vi "ndipolaris Measurement Example.vi"() -> ()   [LabVIEW 2013]
doc: "This example shows how to use the driver's VI's to set up the Polaris and acquire transformations. For this example, all wired tools are activated and one wireless tool is activated."
panel:
  out "Front View (YX)":cluster{dbl, dbl}[](graph)
  out "Left Side View (ZX)":cluster{dbl, dbl}[](graph)
  out "Top View (YZ)":cluster{dbl, dbl}[](graph)
  out "Current Transformations":T1(array[cluster])
  in  "Track Stray Markers? (F:No)":bool
  in  "VISA resource name":refnum<visa-resource-name>="COM1"
  in  "Reset? (T:Yes)":bool=TRUE
  in  "Track Outside Measurement Volume? (F:No)":bool
  in  "Location of ROM File for Tool":path=path "C:/Program Files/Northern Digital Inc/8700248.rom"
  in  "Serial Configuration":T2={"Baud Rate (9600)"=9600, "Flow Control (0:None)"=0, "Parity"=0, "Data Bits"=8, "Stop Bits"=10} {"Stop Bits" items=["1.0"=10, "2.0"=20]; "Parity" items=["None", "Odd", "Even"]; "Flow Control (0:None)" items=["None", "XON/XOFF"]; "Baud Rate (9600)" items=["9600"=9600, "14.4k"=14400, "19.2k"=19200, "38.4k"=38400, "57.6k "=57600, "115.2k"=115200]}
  in  "STOP":bool
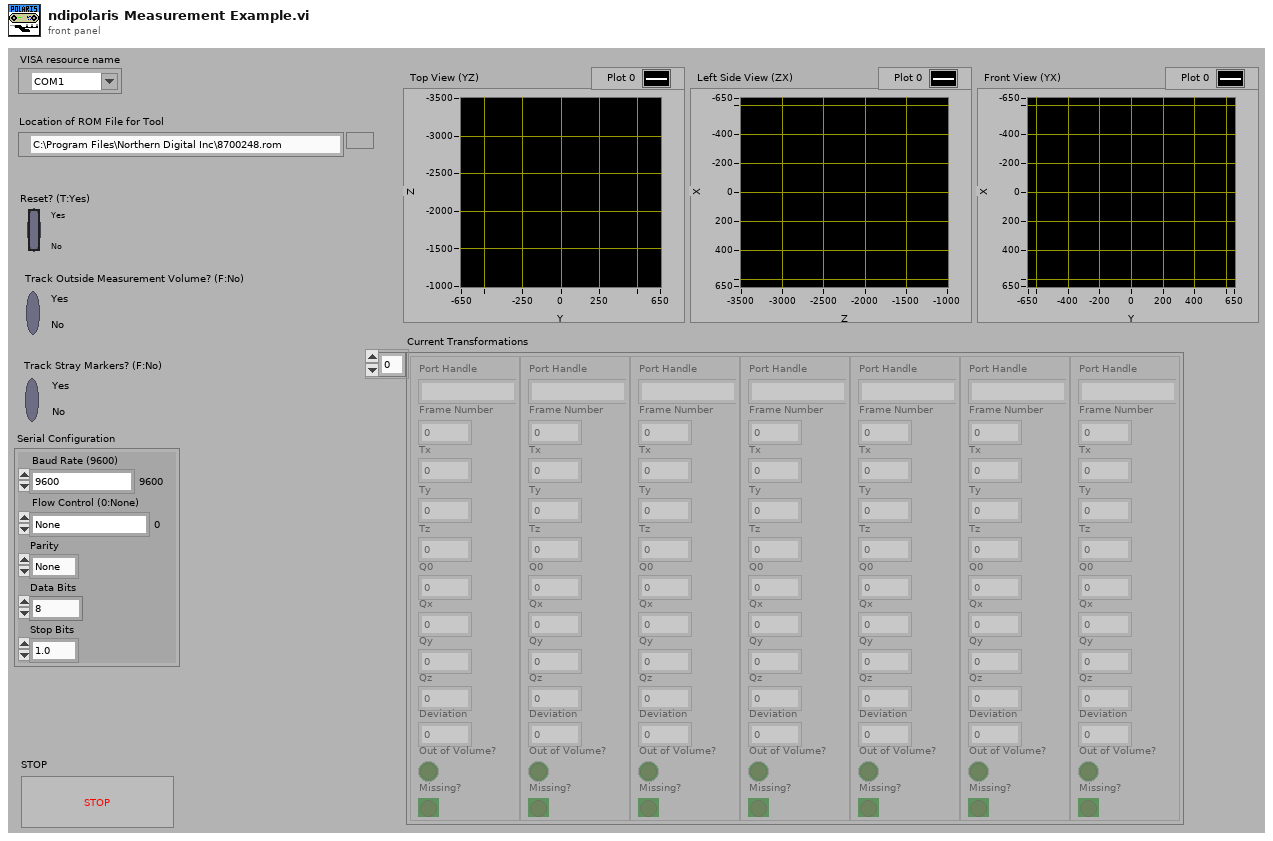
[diagram p1: front panel]
types:
  T1 = cluster{"Port Handle":string, "Frame Number":u32, "Tx":dbl, "Ty":dbl, "Tz":dbl, "Q0":dbl, "Qx":dbl, "Qy":dbl, "Qz":dbl, "Deviation":dbl, "Missing?":bool, "Out of Volume?":bool}[]
  T2 = cluster{"Baud Rate (9600)":u32, "Flow Control (0:None)":u16, "Parity":u16, "Data Bits":u16, "Stop Bits":u16}
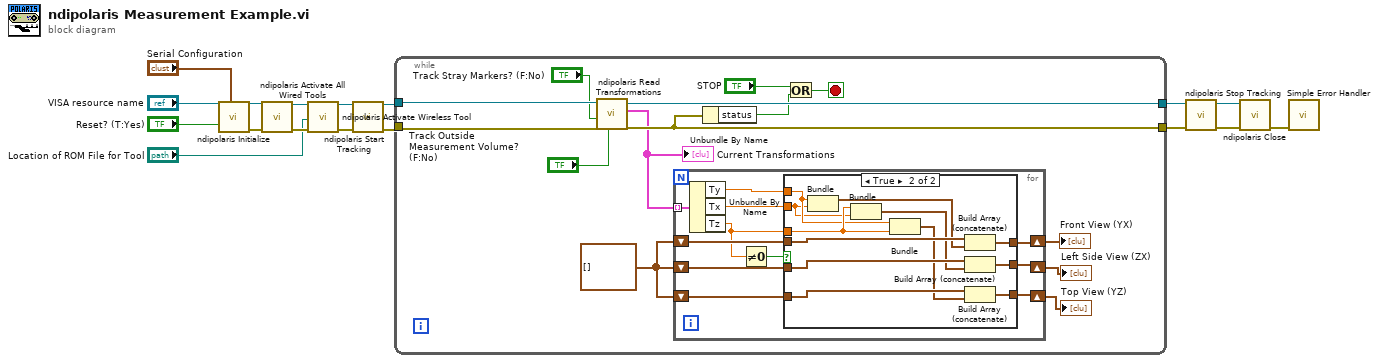
[diagram p0: block diagram]
diagram:
  n1 = call <instrlib>:"ndipolaris Initialize.vi"("Serial Configuration"="Serial Configuration", "Reset? (T: Yes)"="Reset? (T:Yes)", "VISA resource name"="VISA resource name") -> ("error out"=w9:errorcluster, "VISA resource name out"=w10:refnum<visa-resource-name>)  [unwired: 7 in]
  n2 = call <instrlib>:"ndipolaris Activate All Wired Tools.vi"("error in (no error)"=w9, "VISA resource name"=w10) -> ("error out"=w16:errorcluster, "VISA resource out"=w17:refnum<visa-resource-name>)  [unwired: 7 in, 1 out]
  n3 = call <instrlib>:"ndipolaris Activate Wireless Tool.vi"("error in (no error)"=w16, "Location of ROM File for Tool"="Location of ROM File for Tool", "VISA resource name"=w17) -> ("error out"=w13:errorcluster, "VISA resource out"=w14:refnum<visa-resource-name>)  [unwired: 6 in, 1 out]
  n4 = call <instrlib>:"ndipolaris Start Tracking.vi"("error in (no error)"=w13, "VISA resource name"=w14) -> ("error out"=w11:errorcluster, "VISA resource out"=w12:refnum<visa-resource-name>)  [unwired: 8 in]
  n5 = while {
    tunnel: w12 -> [w31]
    tunnel: w11 -> [w30]
    tunnel: [w27] -> w7
    tunnel: [w26] -> w6
    stop <- w29 stop-if-true
    w23 = cluster{dbl, dbl}[] [] ("Top View (YZ)")
    n6 = call <instrlib>:"ndipolaris Read Transformations.vi"("Track Outside Measurement Volume? (F:No)"="Track Outside Measurement Volume? (F:No)", "error in (no error)"=w30, "Track Stray Markers? (F:No)"="Track Stray Markers? (F:No)", "VISA resource name"=w31) -> ("error out"=w26:errorcluster, "Transformations"=w18:T1, "VISA resource out"=w27:refnum<visa-resource-name>)  [unwired: 4 in, 1 out]
    "Current Transformations" <- w18
    n7 = for {
      tunnel: w18 -> [w42] mode=indexing
      shift-right: [w34] -> w20
      shift-left: w23 -> [w39]
      shift-right: [w33] -> w21
      shift-left: w23 -> [w40]
      shift-right: [w32] -> w22
      shift-left: w23 -> [w38]
      n8 = Unbundle By Name(w42) -> ("Ty"=w37:dbl, "Tx"=w36:dbl, "Tz"=w35:dbl)
      n9 = Not Equal To 0?(x=w35) -> (x != 0?=w41:bool)
      n10 = case shown="True" w41 {
        tunnel: w40 -> [w44 w56]
        tunnel: w39 -> [w45 w55]
        tunnel: w38 -> [w43 w57]
        tunnel: w37 -> [_ w47]
        tunnel: w36 -> [_ w46]
        tunnel: w35 -> [_ w48]
        tunnel: [w45 w51] -> w34
        tunnel: [w44 w50] -> w33
        tunnel: [w43 w49] -> w32
        frame False {
        }
        frame True {
          n11 = Bundle("Ty"=w47, "Tx"=w46) -> (w52:cluster{"Ty":dbl, "Tx":dbl})  [unwired: 1 in]
          n12 = Bundle("Tz"=w48, "Tx"=w46) -> (w53:cluster{"Tz":dbl, "Tx":dbl})  [unwired: 1 in]
          n13 = Bundle("Ty"=w47, "Tz"=w48) -> (w54:cluster{"Ty":dbl, "Tz":dbl})  [unwired: 1 in]
          n14 = Build Array (concatenate)(w55, w52) -> (w51:cluster{"Ty":dbl, "Tx":dbl}[])
          n15 = Build Array (concatenate)(w56, w53) -> (w50:cluster{"Tz":dbl, "Tx":dbl}[])
          n16 = Build Array (concatenate)(w57, w54) -> (w49:cluster{"Ty":dbl, "Tz":dbl}[])
        }
      }
    }
    "Left Side View (ZX)" <- w21
    "Top View (YZ)" <- w22
    "Front View (YX)" <- w20
    n17 = Unbundle By Name(w26) -> ("status"=w25:bool)
    n18 = Or(x="STOP", y=w25) -> (x .or. y?=w29:bool)
  }
  n19 = call <instrlib>:"ndipolaris Stop Tracking.vi"("error in (no error)"=w6, "VISA resource name"=w7) -> ("error out"=w3:errorcluster, "VISA resource out"=w4:refnum<visa-resource-name>)  [unwired: 8 in]
  n20 = call <instrlib>:"ndipolaris Close.vi"("error in (no error)"=w3, "VISA resource name"=w4) -> ("error out"=w2:errorcluster)  [unwired: 9 in]
  n21 = call <vilib>:"Simple Error Handler.vi"("error in (no error)"=w2) -> ()  [unwired: 4 in, 5 out]
